vi "Set Current.vi"(8 "error in (no error)":errorcluster, 10 "Current":dbl, 11 "Keysight in":refnum<class "PS Keysight.lvclass">) -> (0 "error out":errorcluster, 3 "Keysight out":refnum<class "PS Keysight.lvclass">)   [LabVIEW 2020, in "PS Keysight.lvclass"]
uses:
  PS Keysight.lvclass
  PS Keysight.lvclass/PS Keysight.ctl
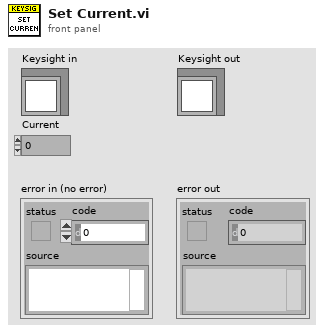
[diagram p1: front panel]
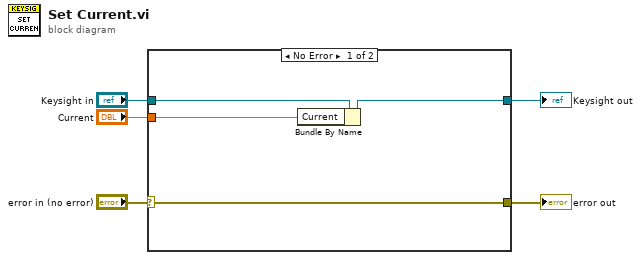
[diagram p0: block diagram]
diagram:
  n1 = case shown="No Error" "error in (no error)" {
    selector: "error in (no error)" -> [w8 w10]
    tunnel: [w7 w11] -> w4
    tunnel: "Keysight in" -> [w9 w11]
    tunnel: [w8 w10] -> w2
    tunnel: "Current" -> [w6 _]
    frame No Error {
      n2 = Bundle By Name(cluster=w9, "Current"=w6) -> (w7:refnum<class "PS Keysight.lvclass">)
    }
    frame Error {
    }
  }
  "error out" <- w2
  "Keysight out" <- w4
